vi "题3.vi"() -> ()   [LabVIEW 2017]
panel:
  out "温度":string
  in  "停止":bool
  in  "温度单位":bool
  out "温度计":dbl(slide) scale=0.0..100.0
  # "℉"
  # "℃"
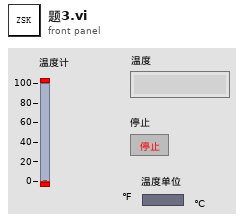
[diagram p1: front panel]
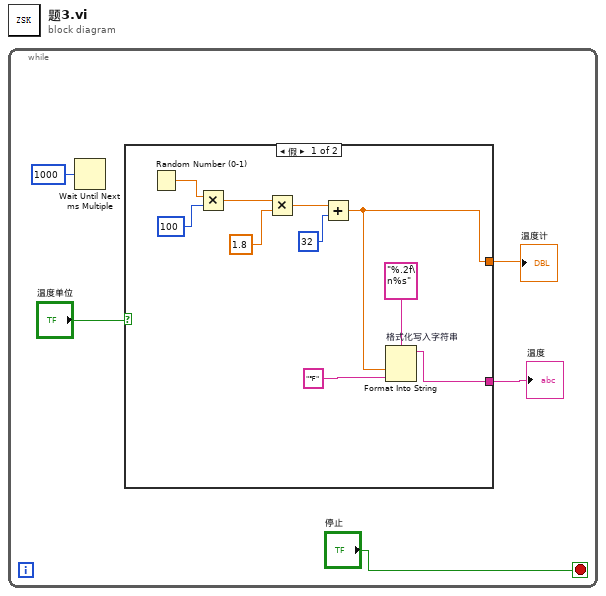
[diagram p0: block diagram]
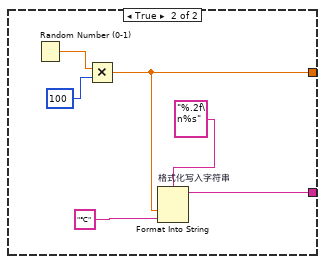
[diagram p2: hidden frame]
diagram:
  n1 = while {
    stop <- "停止" stop-if-true
    n2 = Wait Until Next ms Multiple(millisecond multiple=u32 1000 ("毫秒倍数")) -> ()  [unwired: 1 out]
    n3 = case shown="假" "温度单位" {
      tunnel: [w8 w18] -> w2
      tunnel: [w6 w17] -> w1
      frame False {
        n4 = Random Number (0-1)() -> (number: 0 to 1=w12:dbl)
        n5 = Multiply(x=w12, y=100) -> (x*y=w10:dbl)
        n6 = Multiply(x=w10, y=1.8) -> (x*y=w15:dbl)
        n7 = Add(x=w15, y=32) -> (x+y=w8:dbl)
        n8 = Format Into String "格式化写入字符串"(format string="%.2f\n%s", w8, "℉") -> (resulting string=w6:string)  [unwired: 2 in, 1 out]
      }
      frame True {
        n9 = Random Number (0-1)() -> (number: 0 to 1=w21:dbl)
        n10 = Multiply(x=w21, y=100) -> (x*y=w18:dbl)
        n11 = Format Into String "格式化写入字符串"(format string="%.2f\n%s", w18, "℃") -> (resulting string=w17:string)  [unwired: 2 in, 1 out]
      }
    }
    "温度计" <- w2
    "温度" <- w1
  }
